vi "RebuildBuildSpecs.vi"(9 "PPL Name":string="TopLibrary.lvlibp", 10 "Build Specification Name":string="My Packed Library", 11 "Project Path":path) -> (1 "Error Out":errorcluster)   [LabVIEW 2011]
uses:
  <vilib>/AppBuilder/AB_API/PPL/NI_AB_API_PPL.lvclass
panel:
  in  "Error In":errorcluster
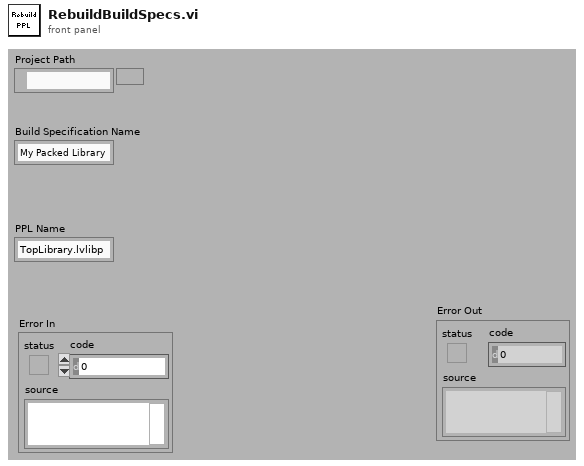
[diagram p1: front panel]
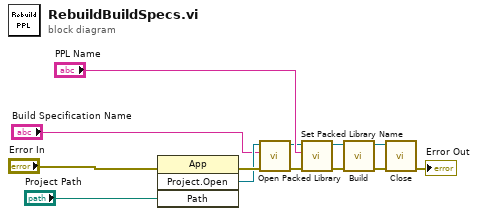
[diagram p0: block diagram]
diagram:
  n1 = invoke class="App" method="Project.Open"(error in="Error In", "Path"="Project Path") -> (error out=w6:errorcluster, "Project:Open"=w5:refnum<vi>)  [unwired: 2 in, 2 out]
  n2 = call <vilib>:"Open Packed Library.vi"("error in (no error)"=w6, "Build specification name"="Build Specification Name", "Project Refnum"=w5) -> ("error out"=w7:errorcluster, "PPL out"=w9:refnum<class "NI_AB_API_PPL.lvclass">)  [unwired: 7 in]
  n3 = call-dynamic "Set Packed Library Name.vi"("error in (no error)"=w7, "Packed library name"="PPL Name", "PPL in"=w9) -> ("error out"=w8:errorcluster, "PPL out"=w10:refnum<class "NI_AB_API_PPL.lvclass">)  [unwired: 7 in]
  n4 = call-dynamic "Build.vi"("error in (no error)"=w8, "PPL in"=w10) -> ("error out"=w12:errorcluster, "PPL out"=w13:refnum<class "NI_AB_API_PPL.lvclass">)  [unwired: 7 in, 1 out]
  n5 = call-dynamic "Close.vi"("error in (no error)"=w12, "DLL in"=w13) -> ("error out"=→"Error Out":errorcluster)  [unwired: 9 in]
